vi "Untitled 4.vi"() -> ()   [LabVIEW 2016]
uses:
  c:/Windows/System32/user32.dll
panel:
  in  "error in":errorcluster
  out "error out":errorcluster
  in  "stop":bool
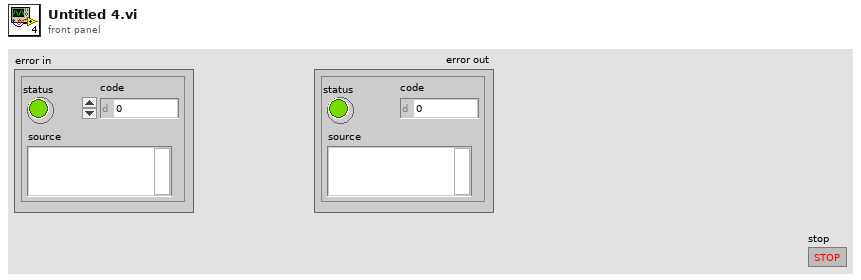
[diagram p1: front panel]
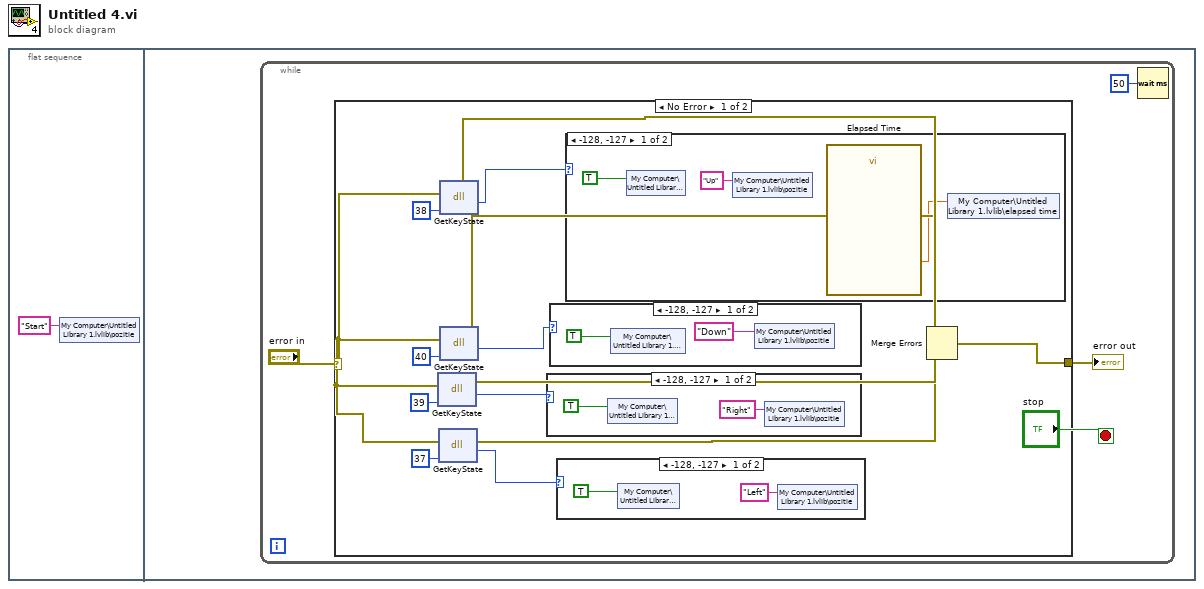
[diagram p0: block diagram]
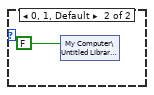
[diagram p2: hidden frame]
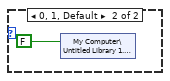
[diagram p3: hidden frame]
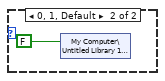
[diagram p4: hidden frame]
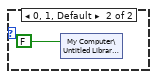
[diagram p5: hidden frame]
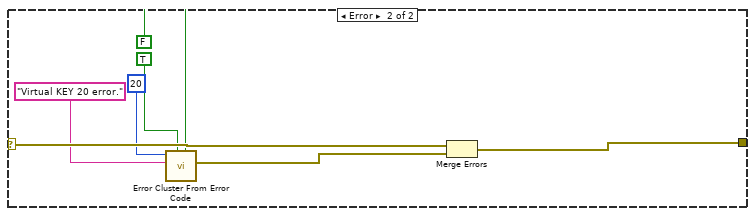
[diagram p6: hidden frame]
diagram:
  n1 = flat-sequence {
    frame #0 {
      n2 = shared-variable "My Computer\\Untitled Library 1.lvlib\\pozitie"("Start" ("pozitie")) -> ()  [unwired: 1 in, 1 out]
    }
    frame #1 {
      n3 = while {
        stop <- "stop" stop-if-true
        n4 = case shown="No Error" "error in" {
          selector: "error in" -> [w19 w38]
          tunnel: [w14 w39] -> w3
          frame No Error {
            n5 = dll-call lib="c:/Windows/System32/User32.dll" fn="GetKeyState"(error in=w19, "nvirtkey"=i16 39) -> (error out=w16:errorcluster, "return type"=w8:i16)  [unwired: 3 in, 1 out]
            n6 = dll-call lib="c:/Windows/System32/User32.dll" fn="GetKeyState"(error in=w19, "nvirtkey"=i16 37) -> (error out=w15:errorcluster, "return type"=w9:i16)  [unwired: 3 in, 1 out]
            n7 = dll-call lib="c:/Windows/System32/User32.dll" fn="GetKeyState"(error in=w19, "nvirtkey"=i16 38) -> (error out=w18:errorcluster, "return type"=w7:i16)  [unwired: 3 in, 1 out]
            n8 = dll-call lib="c:/Windows/System32/User32.dll" fn="GetKeyState"(error in=w19, "nvirtkey"=i16 40) -> (error out=w17:errorcluster, "return type"=w6:i16)  [unwired: 3 in, 1 out]
            n9 = case shown="-128, -127" w8 {
              frame -128, -127 {
                n10 = shared-variable "My Computer\\Untitled Library 1.lvlib\\right"(TRUE) -> ()  [unwired: 1 in, 1 out]
                n11 = shared-variable "My Computer\\Untitled Library 1.lvlib\\pozitie"("Right" ("pozitie")) -> ()  [unwired: 1 in, 1 out]
              }
              frame 0, 1, Default {
                n12 = shared-variable "My Computer\\Untitled Library 1.lvlib\\right"(FALSE) -> ()  [unwired: 1 in, 1 out]
              }
            }
            n13 = case shown="-128, -127" w6 {
              frame -128, -127 {
                n14 = shared-variable "My Computer\\Untitled Library 1.lvlib\\down"(TRUE) -> ()  [unwired: 1 in, 1 out]
                n15 = shared-variable "My Computer\\Untitled Library 1.lvlib\\pozitie"("Down" ("pozitie")) -> ()  [unwired: 1 in, 1 out]
              }
              frame 0, 1, Default {
                n16 = shared-variable "My Computer\\Untitled Library 1.lvlib\\down"(FALSE) -> ()  [unwired: 1 in, 1 out]
              }
            }
            n17 = case shown="-128, -127" w9 {
              frame -128, -127 {
                n18 = shared-variable "My Computer\\Untitled Library 1.lvlib\\left"(TRUE) -> ()  [unwired: 1 in, 1 out]
                n19 = shared-variable "My Computer\\Untitled Library 1.lvlib\\pozitie"("Left" ("pozitie")) -> ()  [unwired: 1 in, 1 out]
              }
              frame 0, 1, Default {
                n20 = shared-variable "My Computer\\Untitled Library 1.lvlib\\left"(FALSE) -> ()  [unwired: 1 in, 1 out]
              }
            }
            n21 = case shown="-128, -127" w7 {
              frame -128, -127 {
                n22 = shared-variable "My Computer\\Untitled Library 1.lvlib\\up"(TRUE) -> ()  [unwired: 1 in, 1 out]
                n23 = shared-variable "My Computer\\Untitled Library 1.lvlib\\pozitie"("Up" ("pozitie")) -> ()  [unwired: 1 in, 1 out]
                n24 = call "Elapsed Time"() -> ("Elapsed Time (s)"=w20:dbl)  [unwired: 12 in, 7 out]
                n25 = shared-variable "My Computer\\Untitled Library 1.lvlib\\elapsed time"(w20) -> ()  [unwired: 1 in, 1 out]
              }
              frame 0, 1, Default {
                n26 = shared-variable "My Computer\\Untitled Library 1.lvlib\\up"(FALSE) -> ()  [unwired: 1 in, 1 out]
              }
            }
            n27 = Merge Errors(w18, w17, w16, w15) -> (w14:errorcluster)
          }
          frame Error {
            n28 = call <vilib>:"Error Cluster From Error Code.vi"("is warning? (False)"=FALSE, "show call chain? (False)"=TRUE, "error message (\"\")"="Virtual KEY 20 error." ("error message (\"\")"), "error code (0)"=20) -> ("error out"=w37:errorcluster)  [unwired: 5 in]
            n29 = Merge Errors(w38, w37) -> (w39:errorcluster)
          }
        }
        "error out" <- w3
        n30 = Wait (ms)(milliseconds to wait=u32 50) -> ()  [unwired: 1 out]
      }
    }
  }
